vi "_Convert Model Name.vi"(2 "Model Name In":T1=enum."IONICS 3Q 210", 3 "Model":string) -> (0 "SingleSource":bool, 1 "Model Name":T1=enum."IONICS 3Q 210")   [LabVIEW 2018]
uses:
  Type/_Instrument Model.ctl
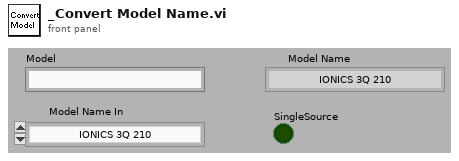
[diagram p1: front panel]
types:
  T1 = typedef "_Instrument Model.ctl" = enum16{"QSight 110", "QSight 120", "QSight 210", "QSight 220", "QSight 410", "QSight 420", "IONICS 3Q 110", "IONICS 3Q 120", "IONICS 3Q 210", "IONICS 3Q 220", "IONICS 3Q 310", "IONICS 3Q 320", "Simulation (Single Source)", "Simulation (Dual Source)"}
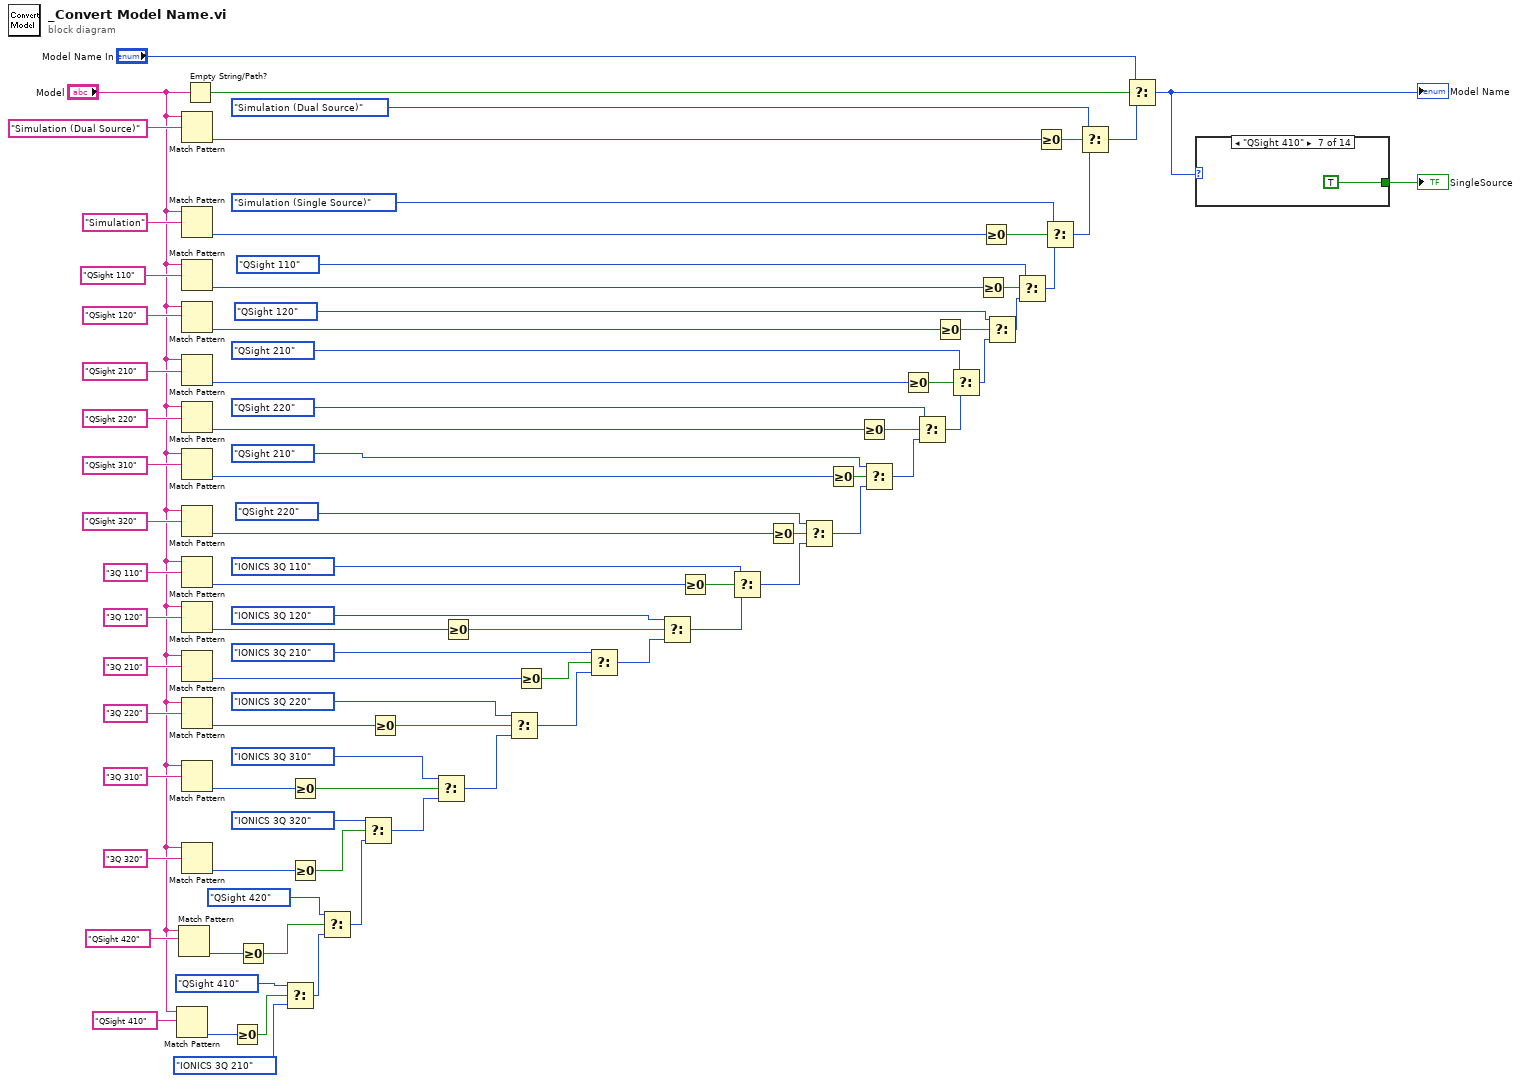
[diagram p0: block diagram]
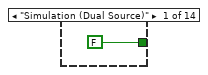
[diagram p2: hidden frame]
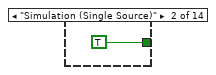
[diagram p3: hidden frame]
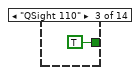
[diagram p4: hidden frame]
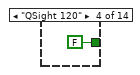
[diagram p5: hidden frame]
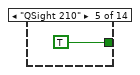
[diagram p6: hidden frame]
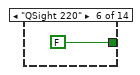
[diagram p7: hidden frame]
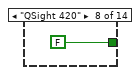
[diagram p8: hidden frame]
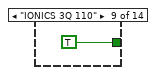
[diagram p9: hidden frame]
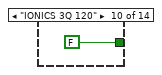
[diagram p10: hidden frame]
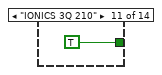
[diagram p11: hidden frame]
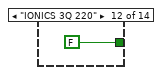
[diagram p12: hidden frame]
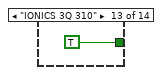
[diagram p13: hidden frame]
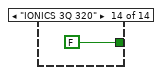
[diagram p14: hidden frame]
diagram:
  n1 = Match Pattern(string="Model", regular expression="QSight 410") -> (offset past match=w8:i32)  [unwired: 4 out]
  n2 = Match Pattern(string="Model", regular expression="QSight 420") -> (offset past match=w9:i32)  [unwired: 4 out]
  n3 = Match Pattern(string="Model", regular expression="Simulation (Dual Source)") -> (offset past match=w84:i32)  [unwired: 4 out]
  n4 = Match Pattern(string="Model", regular expression="Simulation") -> (offset past match=w69:i32)  [unwired: 4 out]
  n5 = Match Pattern(string="Model", regular expression="QSight 110") -> (offset past match=w31:i32)  [unwired: 4 out]
  n6 = Match Pattern(string="Model", regular expression="QSight 120") -> (offset past match=w32:i32)  [unwired: 4 out]
  n7 = Match Pattern(string="Model", regular expression="QSight 210") -> (offset past match=w74:i32)  [unwired: 4 out]
  n8 = Match Pattern(string="Model", regular expression="QSight 220") -> (offset past match=w75:i32)  [unwired: 4 out]
  n9 = Match Pattern(string="Model", regular expression="QSight 310") -> (offset past match=w17:i32)  [unwired: 4 out]
  n10 = Match Pattern(string="Model", regular expression="QSight 320") -> (offset past match=w21:i32)  [unwired: 4 out]
  n11 = Match Pattern(string="Model", regular expression="3Q 110") -> (offset past match=w67:i32)  [unwired: 4 out]
  n12 = Match Pattern(string="Model", regular expression="3Q 120") -> (offset past match=w68:i32)  [unwired: 4 out]
  n13 = Match Pattern(string="Model", regular expression="3Q 210") -> (offset past match=w59:i32)  [unwired: 4 out]
  n14 = Match Pattern(string="Model", regular expression="3Q 220") -> (offset past match=w39:i32)  [unwired: 4 out]
  n15 = Match Pattern(string="Model", regular expression="3Q 310") -> (offset past match=w42:i32)  [unwired: 4 out]
  n16 = Match Pattern(string="Model", regular expression="3Q 320") -> (offset past match=w43:i32)  [unwired: 4 out]
  n17 = Empty String/Path?(string/path="Model") -> (empty?=w50:bool)
  n18 = Greater Or Equal To 0?(x=w8) -> (x >= 0?=w6:bool)
  n19 = Greater Or Equal To 0?(x=w9) -> (x >= 0?=w7:bool)
  n20 = Select(t=_Instrument_Model."QSight 410" ("Model Name"), s=w6, f=_Instrument_Model."IONICS 3Q 210" ("Model Name")) -> (s? t:f=w2:T1)
  n21 = Greater Or Equal To 0?(x=w42) -> (x >= 0?=w41:bool)
  n22 = Greater Or Equal To 0?(x=w43) -> (x >= 0?=w44:bool)
  n23 = Select(t=_Instrument_Model."QSight 420" ("Model Name"), s=w7, f=w2) -> (s? t:f=w5:T1)
  n24 = Select(t=_Instrument_Model."IONICS 3Q 320" ("Model Name"), s=w44, f=w5) -> (s? t:f=w47:T1)
  n25 = Greater Or Equal To 0?(x=w39) -> (x >= 0?=w58:bool)
  n26 = Select(t=_Instrument_Model."IONICS 3Q 310" ("Model Name"), s=w41, f=w47) -> (s? t:f=w37:T1)
  n27 = Greater Or Equal To 0?(x=w68) -> (x >= 0?=w65:bool)
  n28 = Select(t=_Instrument_Model."IONICS 3Q 220" ("Model Name"), s=w58, f=w37) -> (s? t:f=w51:T1)
  n29 = Greater Or Equal To 0?(x=w59) -> (x >= 0?=w60:bool)
  n30 = Select(t=_Instrument_Model."IONICS 3Q 210" ("Model Name"), s=w60, f=w51) -> (s? t:f=w52:T1)
  n31 = Select(t=_Instrument_Model."IONICS 3Q 120" ("Model Name"), s=w65, f=w52) -> (s? t:f=w53:T1)
  n32 = Greater Or Equal To 0?(x=w67) -> (x >= 0?=w66:bool)
  n33 = Select(t=_Instrument_Model."IONICS 3Q 110" ("Model Name"), s=w66, f=w53) -> (s? t:f=w19:T1)
  n34 = Greater Or Equal To 0?(x=w21) -> (x >= 0?=w22:bool)
  n35 = Select(t=_Instrument_Model."QSight 220" ("Model Name"), s=w22, f=w19) -> (s? t:f=w16:T1)
  n36 = Greater Or Equal To 0?(x=w17) -> (x >= 0?=w18:bool)
  n37 = Greater Or Equal To 0?(x=w75) -> (x >= 0?=w76:bool)
  n38 = Select(t=_Instrument_Model."QSight 210" ("Model Name"), s=w18, f=w16) -> (s? t:f=w15:T1)
  n39 = Greater Or Equal To 0?(x=w74) -> (x >= 0?=w73:bool)
  n40 = Select(t=_Instrument_Model."QSight 220" ("Model Name"), s=w76, f=w15) -> (s? t:f=w82:T1)
  n41 = Greater Or Equal To 0?(x=w32) -> (x >= 0?=w29:bool)
  n42 = Select(t=_Instrument_Model."QSight 210" ("Model Name"), s=w73, f=w82) -> (s? t:f=w26:T1)
  n43 = Greater Or Equal To 0?(x=w31) -> (x >= 0?=w30:bool)
  n44 = Greater Or Equal To 0?(x=w69) -> (x >= 0?=w70:bool)
  n45 = Select(t=_Instrument_Model."QSight 120" ("Model Name"), s=w29, f=w26) -> (s? t:f=w25:T1)
  n46 = Select(t=_Instrument_Model."QSight 110" ("Model Name"), s=w30, f=w25) -> (s? t:f=w24:T1)
  n47 = Greater Or Equal To 0?(x=w84) -> (x >= 0?=w83:bool)
  n48 = Select(t=_Instrument_Model."Simulation (Single Source)" ("Model Name"), s=w70, f=w24) -> (s? t:f=w81:T1)
  n49 = Select(t=_Instrument_Model."Simulation (Dual Source)" ("Model Name"), s=w83, f=w81) -> (s? t:f=w48:T1)
  n50 = Select(t="Model Name In", s=w50, f=w48) -> (s? t:f=w36:T1)
  "Model Name" <- w36
  n51 = case shown="\"QSight 410\"" w36 {
    tunnel: [FALSE ("SingleSource") TRUE ("SingleSource") TRUE ("SingleSource") FALSE ("SingleSource") TRUE ("SingleSource") FALSE ("SingleSource") TRUE ("SingleSource") FALSE ("SingleSource") TRUE ("SingleSource") FALSE ("SingleSource") TRUE ("SingleSource") FALSE ("SingleSource") TRUE ("SingleSource") FALSE ("SingleSource")] -> w35
    frame "Simulation (Dual Source)" {
    }
    frame "Simulation (Single Source)" {
    }
    frame "QSight 110" {
    }
    frame "QSight 120" {
    }
    frame "QSight 210" {
    }
    frame "QSight 220" {
    }
    frame "QSight 410" {
    }
    frame "QSight 420" {
    }
    frame "IONICS 3Q 110" {
    }
    frame "IONICS 3Q 120" {
    }
    frame "IONICS 3Q 210" {
    }
    frame "IONICS 3Q 220" {
    }
    frame "IONICS 3Q 310" {
    }
    frame "IONICS 3Q 320" {
    }
  }
  "SingleSource" <- w35
